vi "Stop.vi"(11 "Execute?":bool) -> ()   [LabVIEW 2012]
uses:
  Globals/Useful Values.vi
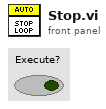
[diagram p1: front panel]
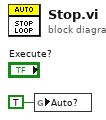
[diagram p0: block diagram]
diagram:
  n1 = global write "Useful Values.vi" "Auto?"(TRUE ("STOP")) -> ()
